vi "Update Obj Position.vi"(8 "error in (no error)":errorcluster, 11 "Pane Object Position in":refnum<class "Pane Object Position.lvclass">) -> (0 "error out":errorcluster, 3 "Pane Object Position out":refnum<class "Pane Object Position.lvclass">)   [LabVIEW 2018, in "Pane Object Position.lvclass"]
uses:
  Pane Object Position.lvclass
  Pane Object Position.lvclass/Pane Object Position.ctl
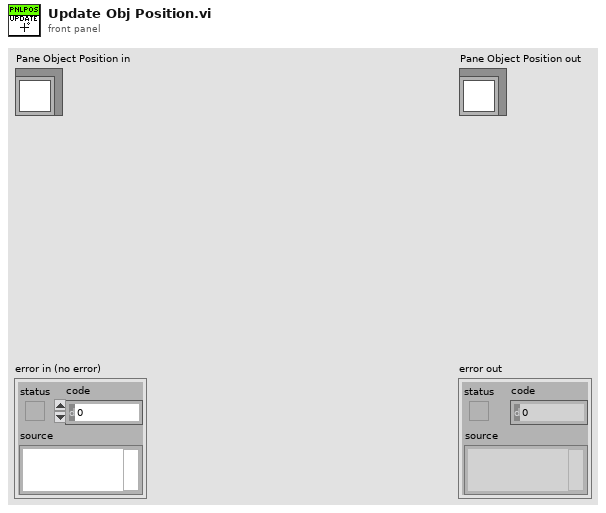
[diagram p1: front panel]
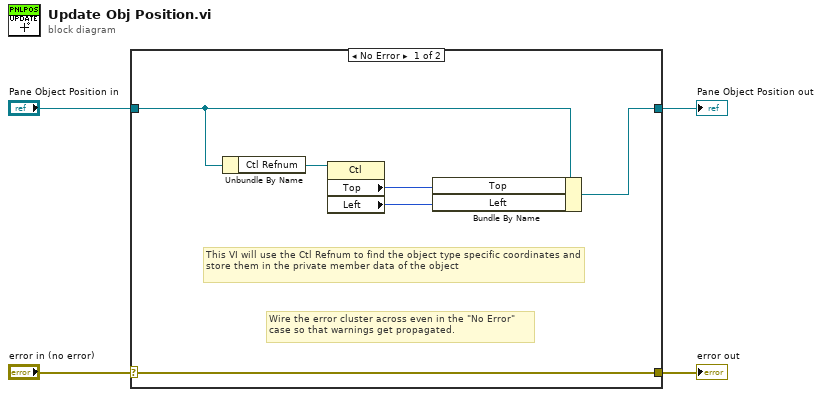
[diagram p0: block diagram]
diagram:
  n1 = case shown="No Error" "error in (no error)" {
    selector: "error in (no error)" -> [w10 w12]
    tunnel: [w10 w12] -> w3
    tunnel: [w7 w11] -> w1
    tunnel: "Pane Object Position in" -> [w8 w11]
    frame No Error {
      # "This VI will use the Ctl Refnum to find the object type specific coordinates and store them in the private member data of the object"
      # "Wire the error cluster across even in the \"No Error\"\ncase so that warnings get propagated."
      n2 = Unbundle By Name(w8) -> ("Ctl Refnum"=w9:refnum<vi>)
      n3 = property class="Ctl"(reference=w9) -> ("Top"=w6:i32, "Left"=w5:i32)  [unwired: 1 in, 2 out]
      n4 = Bundle By Name(cluster=w8, "Top"=w6, "Left"=w5) -> (w7:refnum<class "Pane Object Position.lvclass">)
    }
    frame Error {
    }
  }
  "error out" <- w3
  "Pane Object Position out" <- w1
